vi "1553 Channels to Address Based Handles.vi"(8 "error in":errorcluster, 10 "1553 channels":T6[](array[typedef]), 11 "Ballard MIL-STD 1553 custom device in":T4 format="%.0x") -> (0 "error out":errorcluster, 1 "address based channel handles":T1[](array[typedef]) {"acyclic frame trigger handles"."handle" format="%.0x"; "start stop handles"."stop handle" format="%.0x"; "start stop handles"."start handle" format="%.0x"}, 2 "address based channels":T4[](array[typedef]) format="%.0x", 3 "Ballard MIL-STD 1553 custom device out":T4 format="%.0x")   [LabVIEW 2020, in "Ballard MIL-STD-1553 Engine.lvlib" / "Implementation.lvlib" / "Address Based Execution Unit.lvclass"]
uses:
  Address Based Execution Unit.lvclass
  <vilib>/NI VeriStand/Custom Device API/Custom Device Item Ref.ctl
  Shared/1553 Channel.ctl
  Shared/Address.ctl
  Shared/Message Definition.ctl
  Shared/Message Type.ctl
  Shared/Terminal Endpoint.ctl
  Shared/Parameter Definition.ctl
  1553 Address Based Handles.ctl
  Start Stop Channel Handles.ctl
  Acyclic Frame Trigger Handle.ctl
  <vilib>/NI VeriStand/Custom Device API/Custom Device API.lvlib
  Scripting/Ballard MIL-STD-1553 Scripting.lvlib
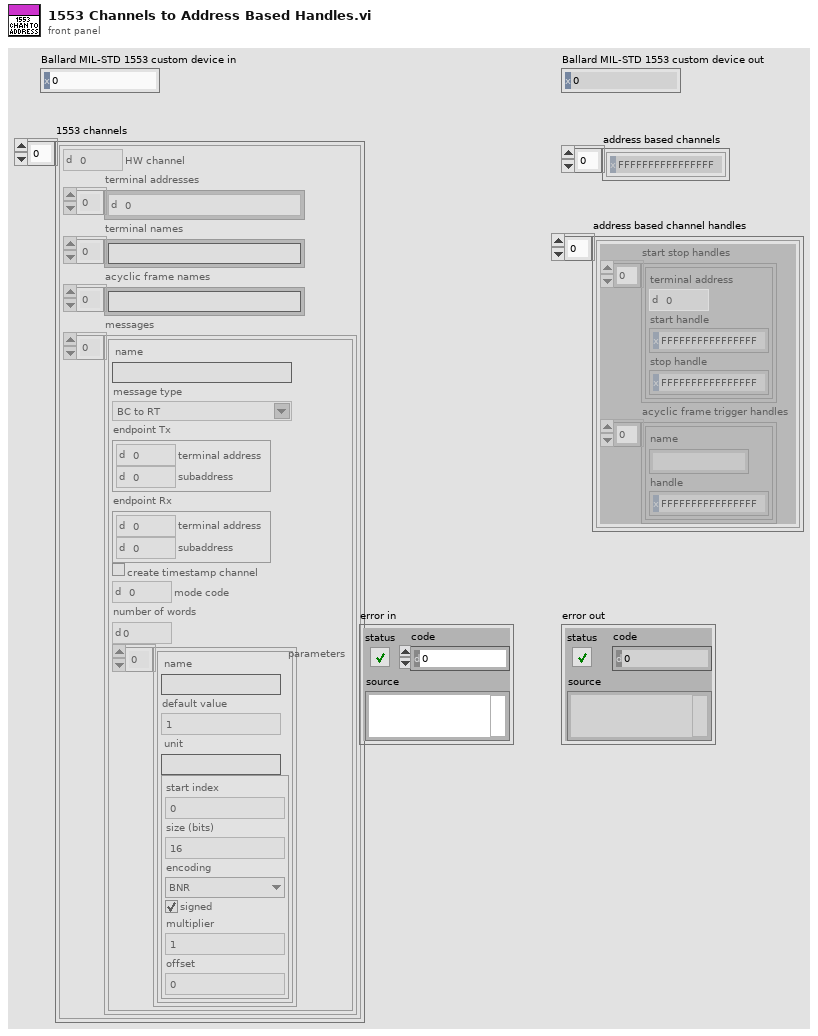
[diagram p1: front panel]
types:
  T1 = typedef "Ballard MIL-STD-1553 Engine.lvlib/Implementation.lvlib/Address Based Execution Unit.lvclass/1553 Address Based Handles.ctl" = cluster{"start stop handles":T2[], "acyclic frame trigger handles":T5[]}
  T2 = typedef "Ballard MIL-STD-1553 Engine.lvlib/Implementation.lvlib/Address Based Execution Unit.lvclass/Start Stop Channel Handles.ctl" = cluster{"terminal address":T3, "start handle":T4, "stop handle":T4}
  T3 = typedef "Address.ctl" = u16
  T4 = typedef "Custom Device API.lvlib/Custom Device Item Ref.ctl" = u64
  T5 = typedef "Ballard MIL-STD-1553 Engine.lvlib/Implementation.lvlib/Address Based Execution Unit.lvclass/Acyclic Frame Trigger Handle.ctl" = cluster{"name":string, "handle":T4}
  T6 = typedef "1553 Channel.ctl" = cluster{"HW channel":u16, "terminal addresses":T3[], "terminal names":string[], "acyclic frame names":string[], "messages":T7[]}
  T7 = typedef "Message Definition.ctl" = cluster{"name":string, "message type":T8, "endpoint Tx":T9, "endpoint Rx":T9, "create timestamp channel":bool, "mode code":u16, "number of words":u16, "parameters":cluster{"name":string, "default value":dbl, "unit":string, "parameter definition":T10}[]}
  T8 = typedef "Message Type.ctl" = string
  T9 = typedef "Terminal Endpoint.ctl" = cluster{"terminal address":T3, "subaddress":T3}
  T10 = typedef "Parameter Definition.ctl" = cluster{"start index":i32, "size (bits)":i32, "encoding":enum16{"BNR", "BCD", "Discrete"}, "signed":bool, "multiplier":dbl, "offset":dbl}
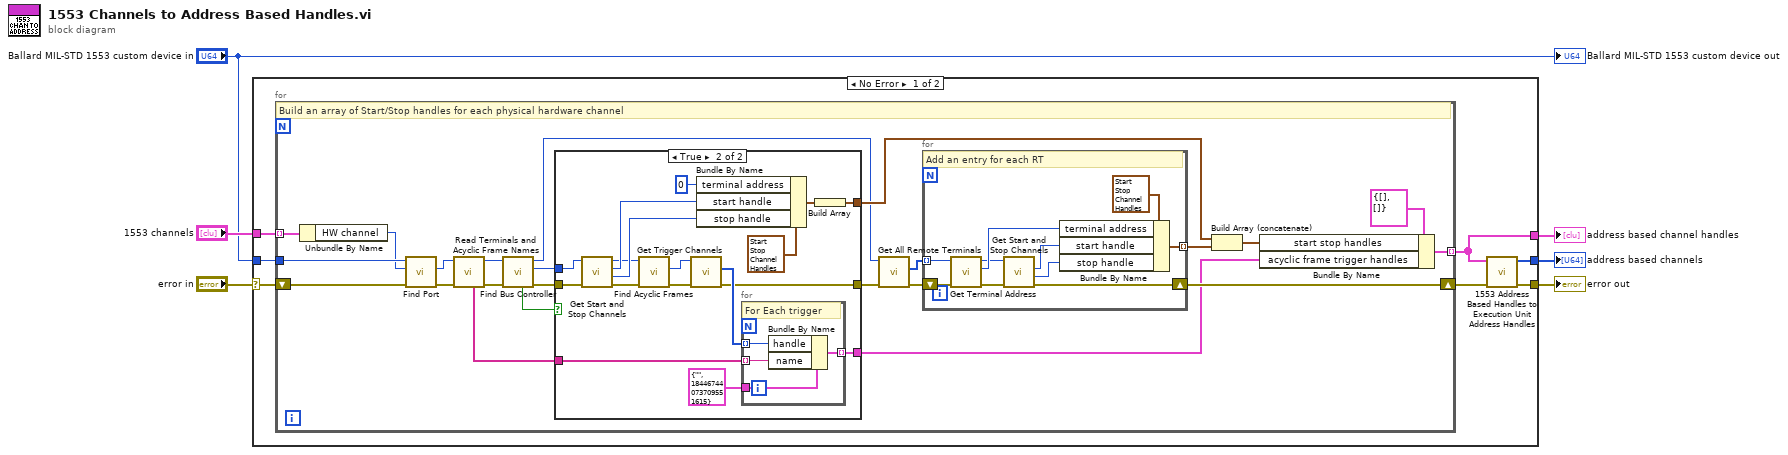
[diagram p0: block diagram]
diagram:
  n1 = case shown="No Error" "error in" {
    selector: "error in" -> [w12 w69]
    tunnel: "1553 channels" -> [w13 _]
    tunnel: "Ballard MIL-STD 1553 custom device in" -> [w11 _]
    tunnel: [w9 w69] -> w4
    tunnel: [w8 _] -> w3
    tunnel: [w7 _] -> w1
    frame No Error {
      n2 = for {
        tunnel: w13 -> [w36] mode=indexing
        shift-right: [w26] -> w10
        shift-left: w12 -> [w35]
        tunnel: w11 -> [w34]
        tunnel: [w21] -> w7 mode=indexing
        # "Build an array of Start/Stop handles for each physical hardware channel"
        n3 = Unbundle By Name(w36) -> ("HW channel"=w33:u16)
        n4 = call "Find Port.vi"("error in"=w35, "port number"=w33, "Ballard MIL-STD 1553 custom device in"=w34) -> ("error out"=w24:errorcluster, "port"=w25:T4)  [unwired: 5 in, 2 out]
        n5 = call "Read Terminals and Acyclic Frame Names.vi"("error in"=w24, "port in"=w25) -> ("error out"=w18:errorcluster, "port out"=w19:T4, "acyclic frame names"=w20:string[])  [unwired: 5 in, 2 out]
        n6 = call "Find Bus Controller.vi"("error in"=w18, "port in"=w19) -> ("error out"=w30:errorcluster, "bus controller"=w23:T4, "port out"=w14:T4, "found?"=w15:bool)  [unwired: 6 in]
        n7 = case shown="True" w15 {
          tunnel: w30 -> [w37 w54]
          tunnel: w23 -> [_ w48]
          tunnel: [_ w45] -> w22
          tunnel: w20 -> [_ w44]
          tunnel: [_ w40] -> w17
          tunnel: [w37 w41] -> w16
          frame False {
          }
          frame True {
            n8 = call "Get Start and Stop Channels.vi"("error in"=w54, "terminal in"=w48) -> ("error out"=w43:errorcluster, "stop channel"=w51:T4, "start channel"=w52:T4, "terminal out"=w42:T4)  [unwired: 5 in, 1 out]
            n9 = call "Find Acyclic Frames.vi"("error in"=w43, "bus controller in"=w42) -> ("error out"=w47:errorcluster, "acyclic frames section"=w49:T4)  [unwired: 6 in, 2 out]
            n10 = call "Get Trigger Channels.vi"("error in"=w47, "acyclic frames section in"=w49) -> ("error out"=w41:errorcluster, "acyclic frame triggers"=w46:T4[])  [unwired: 6 in, 2 out]
            n11 = Bundle By Name(cluster=T2 {"terminal address"=0, "start handle"=18446744073709551615, "stop handle"=18446744073709551615} ("start stop handle"), "terminal address"=T3 0, "start handle"=w52, "stop handle"=w51) -> (w39:T2)
            n12 = for {
              tunnel: w44 -> [w56] mode=indexing
              tunnel: w46 -> [w58] mode=indexing
              tunnel: [w57] -> w45 mode=indexing
              tunnel: T5 {"name"="", "handle"=18446744073709551615} ("acyclic frame trigger handle") -> [w55]
              # "For Each trigger"
              n13 = Bundle By Name(cluster=w55, "handle"=w58, "name"=w56) -> (w57:T5)
            }
            n14 = Build Array(w39) -> (w40:T2[])
          }
        }
        n15 = call "Get All Remote Terminals.vi"("error in"=w16, "port in"=w14) -> ("error out"=w32:errorcluster, "remote terminals"=w31:T4[])  [unwired: 7 in, 1 out]
        n16 = for {
          shift-right: [w60] -> w26
          shift-left: w32 -> [w67]
          tunnel: w31 -> [w66] mode=indexing
          tunnel: [w59] -> w29 mode=indexing
          # "Add an entry for each RT"
          n17 = call "Get Terminal Address.vi"("error in"=w67, "remote terminal in"=w66) -> ("error out"=w64:errorcluster, "terminal address"=w65:T3, "remote terminal out"=w63:T4)  [unwired: 6 in, 1 out]
          n18 = call "Get Start and Stop Channels.vi"("error in"=w64, "terminal in"=w63) -> ("error out"=w60:errorcluster, "stop channel"=w61:T4, "start channel"=w62:T4)  [unwired: 5 in, 2 out]
          n19 = Bundle By Name(cluster=T2 {"terminal address"=0, "start handle"=18446744073709551615, "stop handle"=18446744073709551615} ("start stop handle"), "terminal address"=w65, "start handle"=w62, "stop handle"=w61) -> (w59:T2)
        }
        n20 = Build Array (concatenate)(w17, w29) -> (w27:T2[])
        n21 = Bundle By Name(cluster=T1 {"start stop handles"=[], "acyclic frame trigger handles"=[]} ("1553 start stop handles"), "start stop handles"=w27, "acyclic frame trigger handles"=w22) -> (w21:T1)
      }
      n22 = call "1553 Address Based Handles to Execution Unit Address Handles.vi"("error in"=w10, "1553 address based channel handles"=w7) -> ("error out"=w9:errorcluster, "address based channels"=w8:T4[])  [unwired: 8 in]
    }
    frame Error {
    }
  }
  "error out" <- w4
  "address based channels" <- w3
  "address based channel handles" <- w1
  "Ballard MIL-STD 1553 custom device out" <- "Ballard MIL-STD 1553 custom device in"
